vi "Overwrite-all-variables.vi"(8 "error in (no error)":errorcluster, 10 "Storage vars.":T1, 11 "Storage params. ref. in":refnum<data-value>) -> (0 "error out":errorcluster, 3 "Storage params. ref.":refnum<data-value>)   [LabVIEW 2013, in "CameraVision.lvlib" / "CV-Storage.lvclass"]
uses:
  CV-Storage.lvclass
  Storage-variables.ctl
  UI/Module-states.ctl
  CV-Storage.lvclass/CV-Storage.ctl
  UI/CV-UI.lvclass
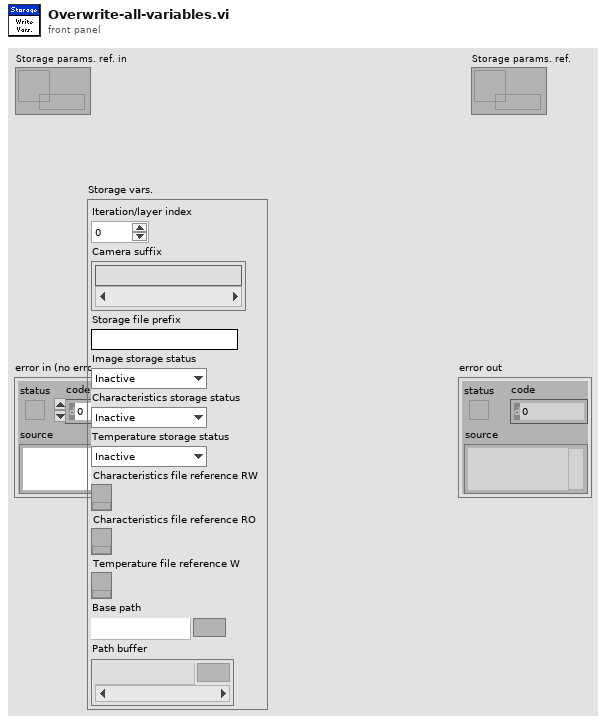
[diagram p1: front panel]
types:
  T1 = typedef "CameraVision.lvlib/CV-Storage.lvclass/Storage-variables.ctl" = cluster{"Iteration/layer index":u16, "Camera suffix":string[], "Storage file prefix":string, "Image storage status":T2, "Characteristics storage status":T2, "Temperature storage status":T2, "Characteristics file reference RW":refnum<k34>, "Characteristics file reference RO":refnum<k34>, "Temperature file reference W":refnum<k34>, "Base path":path, "Path buffer":path[]}
  T2 = typedef "CameraVision.lvlib/CV-UI.lvclass/Module-states.ctl" = enum16{"Inactive", "Active", "Data-loss", "Error", "Simulation", "Synchronizing", "Initialized", "Released"}
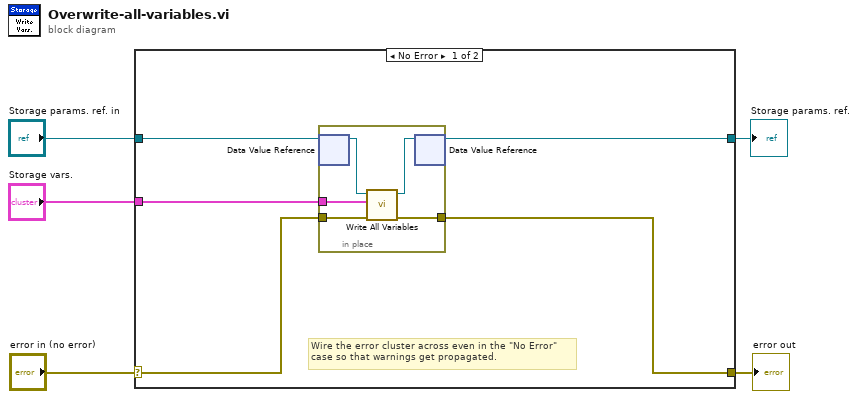
[diagram p0: block diagram]
diagram:
  n1 = case shown="No Error" "error in (no error)" {
    selector: "error in (no error)" -> [w8 w17]
    tunnel: [w9 w17] -> w4
    tunnel: "Storage params. ref. in" -> [w7 w16]
    tunnel: "Storage vars." -> [w10 _]
    tunnel: [w6 w16] -> w1
    frame No Error {
      # "Wire the error cluster across even in the \"No Error\"\ncase so that warnings get propagated."
      n2 = in-place {
        in-place-border: w10 -> [w15]
        in-place-border: [w14] -> w9
        in-place-border: w8 -> [w13]
        n3 = in-place-dvr #1(w7) -> (w12:refnum<class "CV-Storage.lvclass">)  [unwired: 1 out]
        n4 = call "Write All Variables.vi"("error in (no error)"=w13, "Storage vars."=w15, "Storage params in"=w12) -> ("error out"=w14:errorcluster, "Storage params out"=w11:refnum<class "CV-Storage.lvclass">)  [unwired: 7 in]
        n5 = in-place-dvr #1(w11) -> (w6:refnum<data-value>)  [unwired: 1 out]
      }
    }
    frame Error {
    }
  }
  "error out" <- w4
  "Storage params. ref." <- w1
